vi "TCP Trick.vi"(8 "error in (no error)":errorcluster, 10 "DAQ Address":cluster{"Port":u16, "Path":string}, 11 "DAQ Sender in":refnum<class "DAQ Sender.lvclass">) -> (0 "error out":errorcluster, 3 "DAQ Sender out":refnum<class "DAQ Sender.lvclass">)   [LabVIEW 2020, in "DAQ Sender.lvlib" / "DAQ Sender.lvclass"]
uses:
  DAQ Sender.lvclass
  DAQ Sender.lvclass/DAQ Sender.ctl
  Ancestor/Ancestor/Ancestor.lvclass/Ancestor.ctl
  Support VIs/Generate Error.vi
  FGV/Error Memory/Get Error Description.vi
  Support VIs/Get PC name.vi
  Ancestor/Ancestor/Read ID.vi
  Support VIs/Get Class Name.vi
  FGV/Error Memory/Error Memory Core.vi
  <vilib>/AdvancedString/Delimited String to 1D String Array.vi
  Support VIs/Circus Root Path.vi
  FGV/Error Memory/Error Crt Lvl checker.vi
  FGV/Error Memory/Error Memory Core.vi/40c8088d-b597-4017-91af-faa98e00292e.vi
  FGV/Error Memory/Error Memory Core.vi/d4a3ab98-063c-4e44-b43d-fbdcfe6c2be2.vi
  Support VIs/Global Memory.vi
  <vilib>/Utility/LVClass/Get LV Class Name.vi
  Support VIs/Is in Packed Library.vi
  Support VIs/TALOS Root path.vi
  Support VIs/Read CSV worksheet.vi
  Support VIs/Global Constants.vi
  <vilib>/Utility/error.llb/General Error Handler.vi
  Support VIs/Error Log.vi
  Ancestor/Ancestor/Ancestor.lvclass
  <vilib>/Comparison/Equal/Equal Functor/Equal Functor.lvclass
  TALOS.lvlib
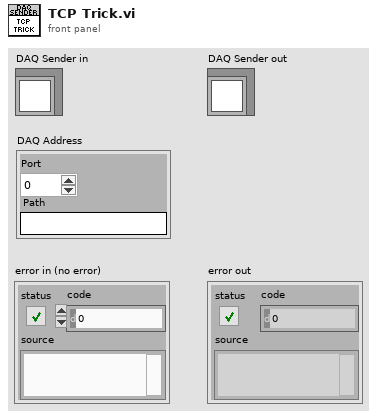
[diagram p1: front panel]
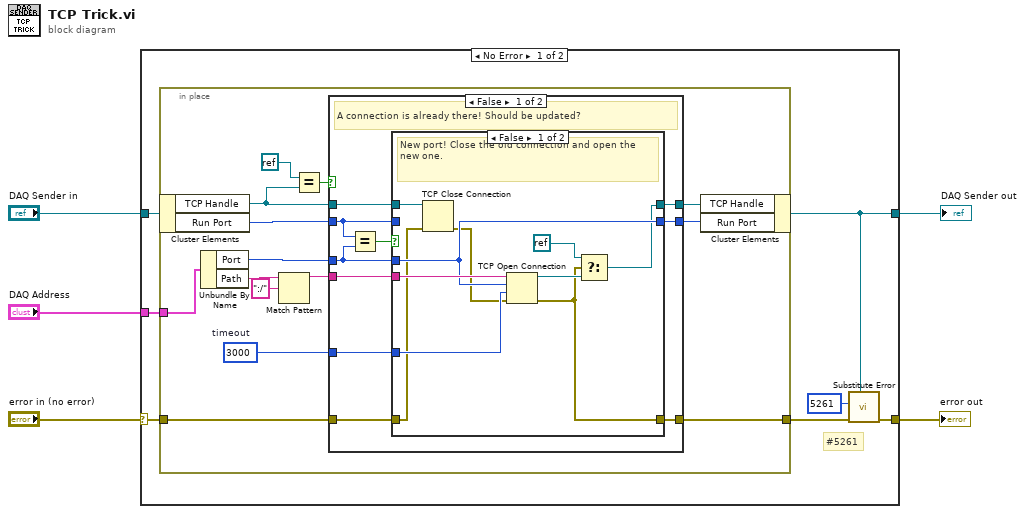
[diagram p0: block diagram]
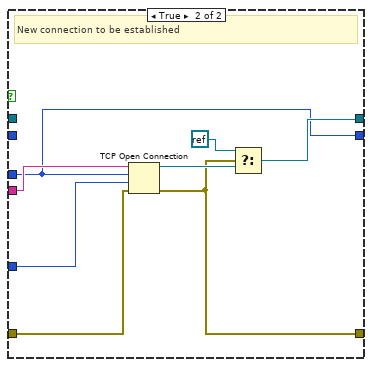
[diagram p3: hidden frame]
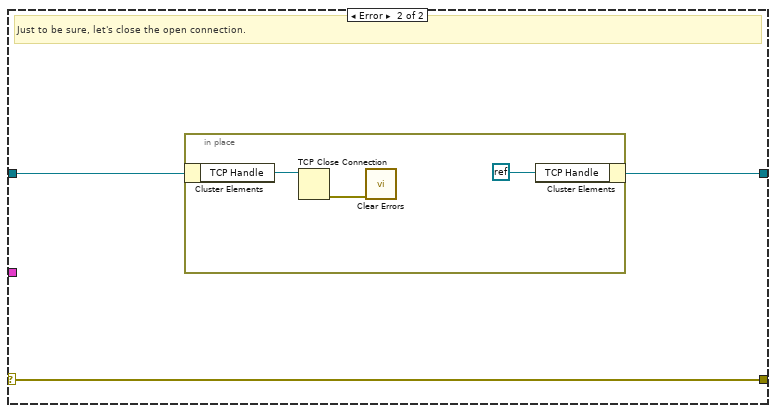
[diagram p4: hidden frame]
diagram:
  n1 = case shown="No Error" "error in (no error)" {
    selector: "error in (no error)" -> [w10 w60]
    tunnel: "DAQ Sender in" -> [w12 w59]
    tunnel: "DAQ Address" -> [w11 _]
    tunnel: [w7 w58] -> w2
    tunnel: [w8 w60] -> w1
    frame No Error {
      # "#5261"
      n2 = in-place {
        in-place-border: w11 -> [w25]
        in-place-border: w10 -> [w19]
        in-place-border: [w17] -> w6
        w13 = 3000  # timeout
        n3 = in-place-cluster #1(w12) -> ("TCP Handle"=w15:refnum<k5>, "Run Port"=w18:u16)
        n4 = Unbundle By Name(w25) -> ("Port"=w20:u16, "Path"=w22:string)
        n5 = Match Pattern(string=w22, regular expression=":/") -> (before substring=w21:string)  [unwired: 1 in, 3 out]
        n6 = Equal?(x=refnum<k0> refnum, y=w15) -> (x = y?=w24:bool)
        n7 = case shown="False" w24 {
          tunnel: w21 -> [w30 w57]
          tunnel: w20 -> [w29 w51]
          tunnel: w19 -> [w36 w56]
          tunnel: [w33 w53] -> w14
          tunnel: w18 -> [w32 _]
          tunnel: [w27 w52] -> w17
          tunnel: [w31 w51] -> w16
          tunnel: w15 -> [w34 _]
          tunnel: w13 -> [w28 w50]
          frame False {
            # "A connection is already there! Should be updated?"
            n8 = Equal?(x=w32, y=w29) -> (x = y?=w35:bool)
            n9 = case shown="False" w35 {
              tunnel: w36 -> [w42 w47]
              tunnel: w34 -> [w46 w49]
              tunnel: [w38 w49] -> w33
              tunnel: w32 -> [_ w48]
              tunnel: [w44 w48] -> w31
              tunnel: w30 -> [w45 _]
              tunnel: w29 -> [w44 _]
              tunnel: w28 -> [w43 _]
              tunnel: [w37 w47] -> w27
              frame False {
                # "New port! Close the old connection and open the new one."
                n10 = TCP Close Connection(connection ID=w46, error in (no error)=w42) -> (error out=w41:errorcluster)  [unwired: 1 in, 1 out]
                n11 = TCP Open Connection(address=w45, remote port or service name=w44, timeout ms (60000)=w43, error in (no error)=w41) -> (connection ID=w40:refnum<k5>, error out=w37:errorcluster)  [unwired: 1 in]
                n12 = Select(t=refnum<k0> refnum, s=w37, f=w40) -> (s? t:f=w38:refnum<k5>)
              }
              frame True {
                # "Still on the same port, do nothing."
              }
            }
          }
          frame True {
            # "New connection to be established"
            n13 = TCP Open Connection(address=w57, remote port or service name=w51, timeout ms (60000)=w50, error in (no error)=w56) -> (connection ID=w54:refnum<k5>, error out=w52:errorcluster)  [unwired: 1 in]
            n14 = Select(t=refnum<k0> refnum, s=w52, f=w54) -> (s? t:f=w53:refnum<k5>)
          }
        }
        n15 = in-place-cluster #1("TCP Handle"=w14, "Run Port"=w16) -> (w7:refnum<class "DAQ Sender.lvclass">)
      }
      n16 = call "Substitute Error.vi"("LabVIEW Object"=w7, "error in (no error)"=w6, "Error Code"=5261) -> ("error out"=w8:errorcluster)  [unwired: 8 in]
    }
    frame Error {
      # "Just to be sure, let's close the open connection."
      n17 = in-place {
        n18 = in-place-cluster #2(w59) -> ("TCP Handle"=w63:refnum<k5>)
        n19 = TCP Close Connection(connection ID=w63) -> (error out=w62:errorcluster)  [unwired: 2 in, 1 out]
        n20 = call <vilib>:"Clear Errors.vi"("error in (no error)"=w62) -> ()  [unwired: 5 in, 2 out]
        n21 = in-place-cluster #2("TCP Handle"=refnum<k0> refnum) -> (w58:refnum<class "DAQ Sender.lvclass">)
      }
    }
  }
  "DAQ Sender out" <- w2
  "error out" <- w1
